vi "SymmetricFunc.vi"(0 "Y":dbl[](array[numeric]), 1 "X":dbl[](array[numeric]), 2 "Coefficients":dbl[](array[numeric])) -> (3 "Y converted":dbl[](array[numeric]), 4 "X converted":dbl[](array[numeric]), 5 "Residue":dbl[](array[numeric]), 6 "f(X,a)":dbl[](array[numeric]))   [LabVIEW 2020, in "XYcenter.lvlib"]
uses:
  XYcenter.lvlib
panel:
  out "data and fit":cluster{dbl[], "Best Polynomial Fit":dbl[]}[](graph)
  out "error out":errorcluster
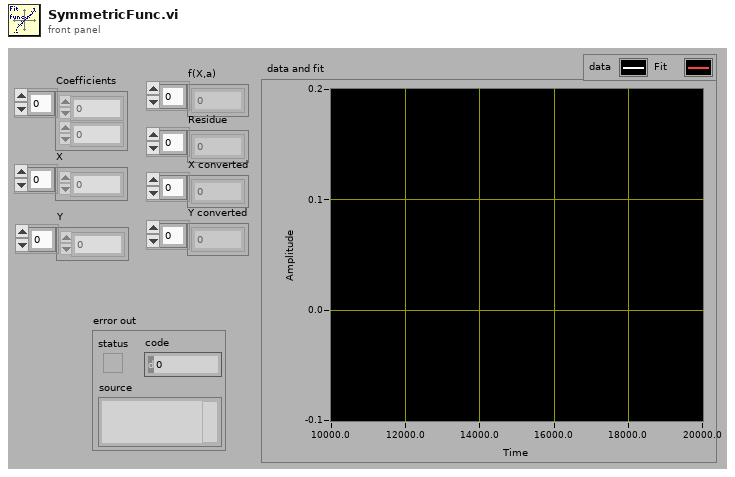
[diagram p1: front panel]
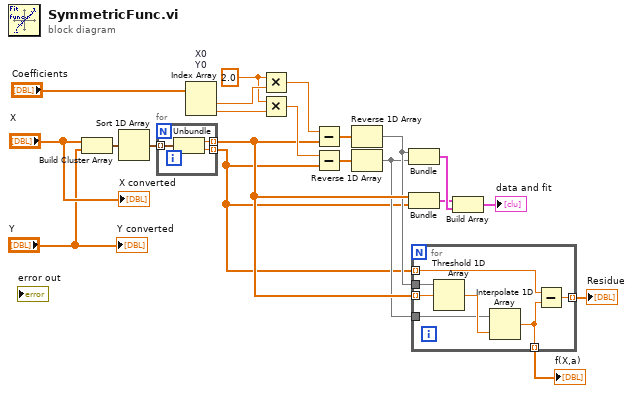
[diagram p0: block diagram]
diagram:
  w20 = 2.0 ("y")
  n1 = Build Cluster Array("X", "Y") -> (w13:cluster{"x":dbl, "x":dbl}[])
  n2 = Sort 1D Array(array=w13) -> (sorted array=w12:cluster{"x":dbl, "x":dbl}[])
  n3 = for {
    tunnel: w12 -> [w24] mode=indexing
    tunnel: [w23] -> w4 mode=indexing
    tunnel: [w22] -> w1 mode=indexing
    n4 = Unbundle(w24) -> ("x"=w23:dbl, "x"=w22:dbl)
  }
  n5 = Index Array "X0\nY0"(array="Coefficients") -> (element #1=w21:dbl, element #2=w19:dbl)  [unwired: 2 in]
  n6 = Multiply(x=w20, y=w21) -> (x*y=w18:dbl)
  n7 = Multiply(x=w20, y=w19) -> (x*y=w17:dbl)
  n8 = Subtract(x=w18, y=w4) -> (x-y=w11:dbl[])
  n9 = Subtract(x=w17, y=w1) -> (x-y=w10:dbl[])
  n10 = Reverse 1D Array(array=w11) -> (reversed array=w3:dbl[])
  n11 = Reverse 1D Array(array=w10) -> (reversed array=w2:dbl[])
  n12 = Bundle(w3, w2) -> (w16:cluster{dbl[], dbl[]})  [unwired: 1 in]
  n13 = Bundle(w4, w1) -> (w15:cluster{dbl[], dbl[]})  [unwired: 1 in]
  n14 = for {
    tunnel: w3 -> [w31]
    tunnel: w2 -> [w29]
    tunnel: w4 -> [w28] mode=indexing
    tunnel: w1 -> [w27] mode=indexing
    tunnel: [w26] -> w6 mode=indexing
    tunnel: [w25] -> w5 mode=indexing
    n15 = Threshold 1D Array(2:w28, 3:w31) -> (0:w30:dbl)  [unwired: 1 in]
    n16 = Interpolate 1D Array(1:w30, 2:w29) -> (0:w25:dbl)
    n17 = Subtract(x=w27, y=w25) -> (x-y=w26:dbl)
  }
  "f(X,a)" <- w5
  "Residue" <- w6
  n18 = Build Array(w15, w16) -> (→"data and fit":cluster{dbl[], dbl[]}[])
  "X converted" <- "X"
  "Y converted" <- "Y"
